vi "DBL to Result.vi"(8 "error in (no error)":errorcluster, 10 "Data":dbl, 11 "Name":string) -> (0 "error out":errorcluster, 3 "Mag Lab Result out":refnum<class "Mag Lab Result.lvclass">)   [LabVIEW 2015]
uses:
  Mag Lab Result.lvclass
  1D wfm (DBL) Result/1D wfm (DBL) Result.lvclass
  Mag Lab Result.lvclass/Mag Lab Result.ctl
  1D wfm (DBL) Result/1D wfm (DBL) Result.lvclass/1D wfm (DBL) Result.ctl
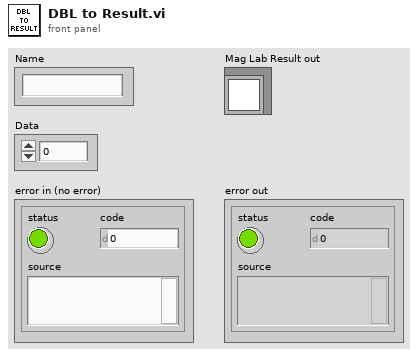
[diagram p1: front panel]
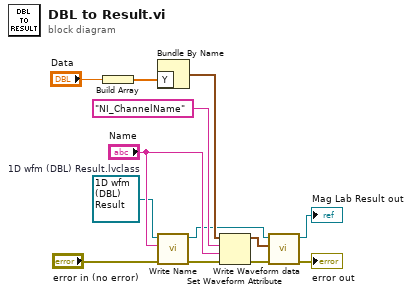
[diagram p0: block diagram]
diagram:
  w6 = refnum<class "1D wfm (DBL) Result.lvclass"> refnum  # 1D wfm (DBL) Result.lvclass
  n1 = Build Array("Data") -> (w7:dbl[])
  n2 = Bundle By Name("Y"=w7) -> (w9:waveform(dbl))  [unwired: 1 in]
  n3 = call "Write Name.vi"("error in (no error)"="error in (no error)", "Name"="Name", "Mag Lab Result in"=w6) -> ("error out"=w12:errorcluster, "Mag Lab Result out"=w5:refnum<class "1D wfm (DBL) Result.lvclass">)  [unwired: 7 in]
  n4 = Set Waveform Attribute(4:w12, 5:"Name", 6:"NI_ChannelName", 7:w9) -> (0:w3:errorcluster, 3:w4:waveform(dbl))  [unwired: 1 out]
  n5 = call "Write Waveform data.vi"("error in (no error)"=w3, "Waveform data"=w4, "1D wfm (DBL) Result in"=w5) -> ("error out"=→"error out":errorcluster, "1D wfm (DBL) Result out"=→"Mag Lab Result out":refnum<class "1D wfm (DBL) Result.lvclass">)  [unwired: 7 in]
